vi "prompt_with_timeout_launcher_v1.0.vi"(8 "error in (no error)":errorcluster, 9 "timer(sec)":i32, 10 "message in":string, 11 "title in":string) -> (0 "error out":errorcluster)   [LabVIEW 2025]
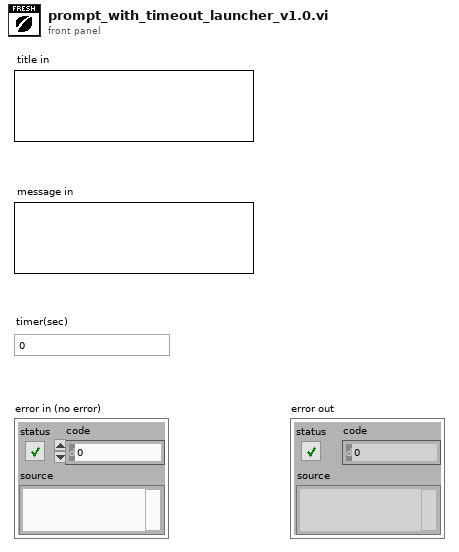
[diagram p1: front panel]
types:
  T1 = enum32{"Invalid", "Standard", "Closed", "Hidden", "Minimized", "Maximized"}
  T2 = enum32{"Bad", "Idle", "Run top level", "Running"}
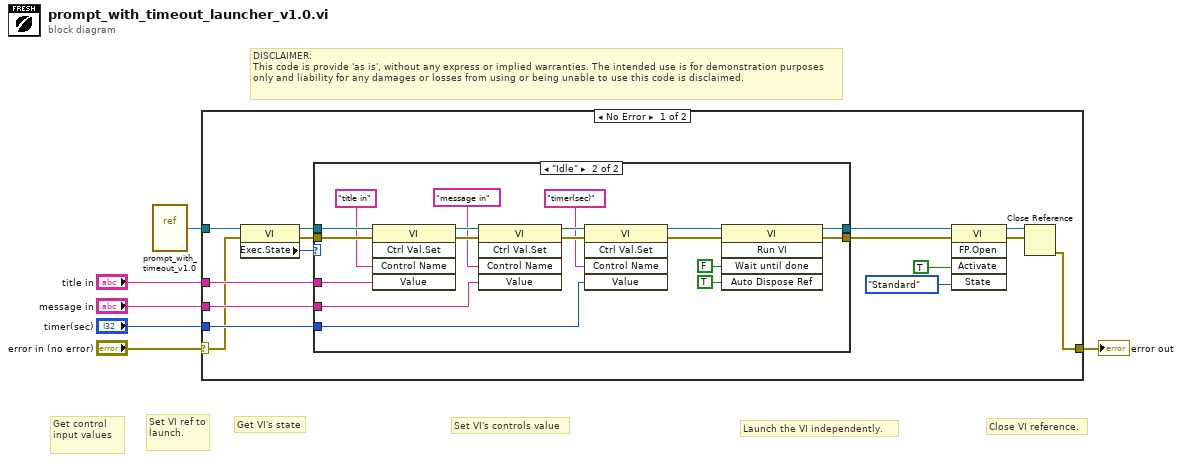
[diagram p0: block diagram]
diagram:
  # "Close VI reference."
  # "Launch the VI independently."
  # "Set VI's controls value"
  # "Get VI's state"
  # "Set VI ref to launch."
  # "Get control input values"
  # "DISCLAIMER:\nThis code is provide 'as is', without any express or implied warranties. The intended use is for demonstration purposes only and liability for any damages or losses from using or being unable to use this code is disclaimed."
  n1 = vi-ref "prompt_with_timeout_v1.0.vi"() -> (w6:refnum<vi>)
  n2 = case shown="No Error" "error in (no error)" {
    selector: "error in (no error)" -> [w14 w42]
    tunnel: w6 -> [w13 _]
    tunnel: [w18 w42] -> w4
    tunnel: "title in" -> [w17 _]
    tunnel: "message in" -> [w16 _]
    tunnel: "timer(sec)" -> [w15 _]
    frame No Error {
      n3 = property class="VI"(reference=w13, error in=w14) -> (reference out=w20:refnum<vi>, error out=w19:errorcluster, "Exec.State"=w21:T2)
      n4 = case shown="\"Idle\"" w21 {
        tunnel: w20 -> [w22 w35]
        tunnel: w19 -> [w23 w39]
        tunnel: [w22 w25] -> w10
        tunnel: [w23 w24] -> w7
        tunnel: w17 -> [_ w28]
        tunnel: w16 -> [_ w27]
        tunnel: w15 -> [_ w26]
        frame Default {
        }
        frame "Idle" {
          n5 = invoke class="VI" method="Ctrl Val.Set"(reference=w35, error in=w39, "Control Name"="title in", "Value"=w28) -> (reference out=w34:refnum<vi>, error out=w38:errorcluster)  [unwired: 1 in, 3 out]
          n6 = invoke class="VI" method="Ctrl Val.Set"(reference=w34, error in=w38, "Control Name"="message in", "Value"=w27) -> (reference out=w33:refnum<vi>, error out=w37:errorcluster)  [unwired: 1 in, 3 out]
          n7 = invoke class="VI" method="Ctrl Val.Set"(reference=w33, error in=w37, "Control Name"="timer(sec)", "Value"=w26) -> (reference out=w32:refnum<vi>, error out=w36:errorcluster)  [unwired: 1 in, 3 out]
          n8 = invoke class="VI" method="Run VI"(reference=w32, error in=w36, "Wait until done"=FALSE ("Wait Until Done"), "Auto Dispose Ref"=TRUE ("Auto Dispose Reference")) -> (reference out=w25:refnum<vi>, error out=w24:errorcluster)  [unwired: 1 in, 3 out]
        }
      }
      n9 = invoke class="VI" method="FP.Open"(reference=w10, error in=w7, "Activate"=TRUE ("Activate?"), "State"=T1."Standard") -> (reference out=w9:refnum<vi>, error out=w8:errorcluster)  [unwired: 1 in, 3 out]
      n10 = Close Reference(reference=w9, error in (no error)=w8) -> (error out=w18:errorcluster)
    }
    frame Error {
    }
  }
  "error out" <- w4
